vi "table_delete_subtable_item.vi"(7 "subtables":string[](array[string]), 8 "error in (no error)":errorcluster, 10 "subkeys":string[](array[string]), 11 "Table in":refnum<class "Table.lvclass">) -> (0 "error out":errorcluster, 2 "found?":bool, 3 "Table out":refnum<class "Table.lvclass">)   [LabVIEW 2020, in "toml.lvclass"]
uses:
  toml.lvclass
  Table/Table.lvclass
  toml.lvclass/toml.ctl
  Item/Item.lvclass
  InlineTable/InlineTable.lvclass
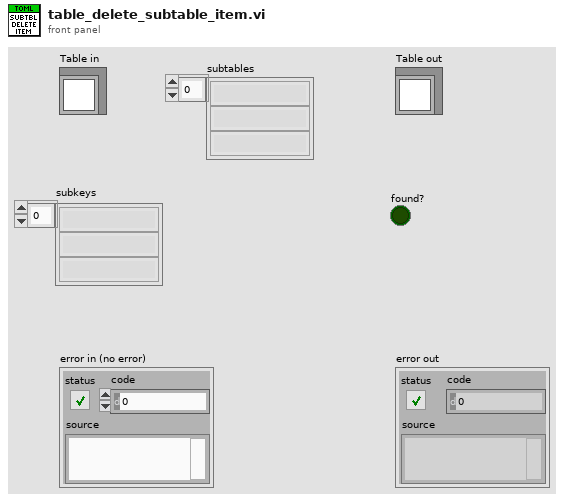
[diagram p1: front panel]
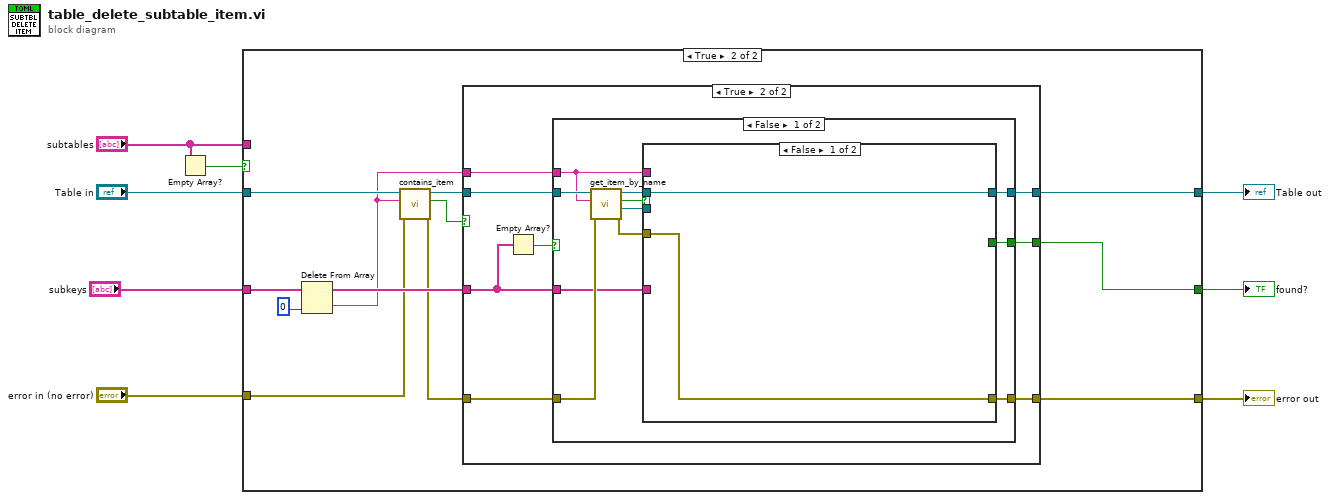
[diagram p0: block diagram]
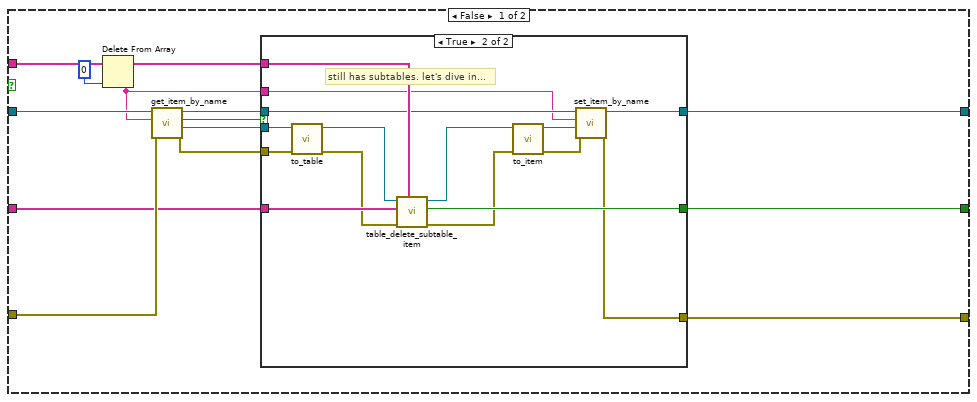
[diagram p2: hidden frame]
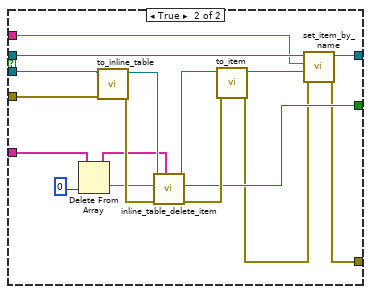
[diagram p5: hidden frame]
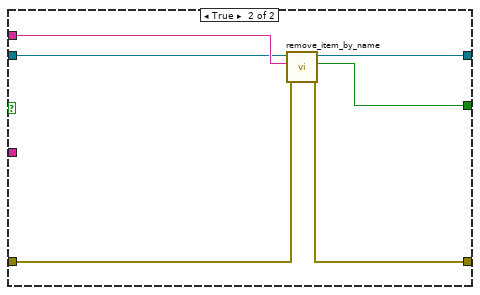
[diagram p6: hidden frame]
diagram:
  n1 = Empty Array?(array="subtables") -> (empty?=w3:bool)
  n2 = case shown="True" w3 {
    tunnel: [w10 w46] -> w8
    tunnel: "subkeys" -> [w15 w49]
    tunnel: [w12 w48] -> w6
    tunnel: "Table in" -> [w19 w44]
    tunnel: "error in (no error)" -> [w18 w42]
    tunnel: "subtables" -> [w22 _]
    tunnel: [w14 w51] -> w1
    frame False {
      n3 = Delete From Array(array=w22, index=0) -> (deleted portion=w11:string, array with subset deleted=w20:string[])  [unwired: 1 in]
      n4 = call "get_item_by_name.vi"("error in (no error)"=w18, "item_name"=w11, "Table in"=w19) -> ("error out"=w16:errorcluster, "Item"=w17:refnum<class "Item.lvclass">, "found?"=w9:bool, "Table out"=w13:refnum<class "Table.lvclass">)  [unwired: 4 in, 1 out]
      n5 = case shown="True" w9 {
        tunnel: w20 -> [_ w39]
        tunnel: w17 -> [_ w38]
        tunnel: w16 -> [w23 w37]
        tunnel: w15 -> [_ w36]
        tunnel: [_ w33] -> w14
        tunnel: w13 -> [w24 w32]
        tunnel: [w24 w31] -> w12
        tunnel: w11 -> [_ w30]
        tunnel: [w23 w25] -> w10
        frame False {
        }
        frame True {
          # "still has subtables. let's dive in..."
          n6 = call "to_table.vi"("error in (no error)"=w37, "Item in"=w38) -> ("error out"=w35:errorcluster, "Table"=w34:refnum<class "Table.lvclass">)  [unwired: 8 in]
          n7 = call "table_delete_subtable_item.vi"("subtables"=w39, "error in (no error)"=w35, "subkeys"=w36, "Table in"=w34) -> ("error out"=w29:errorcluster, "found?"=w33:bool, "Table out"=w28:refnum<class "Table.lvclass">)  [unwired: 5 in]
          n8 = call "to_item.vi"("error in (no error)"=w29, "Table in"=w28) -> ("error out"=w26:errorcluster, "Item out"=w27:refnum<class "Item.lvclass">)  [unwired: 8 in]
          n9 = call "set_item_by_name.vi"("error in (no error)"=w26, "Item"=w27, "item_name"=w30, "Table in"=w32) -> ("error out"=w25:errorcluster, "Table out"=w31:refnum<class "Table.lvclass">)  [unwired: 6 in]
        }
      }
    }
    frame True {
      n10 = Delete From Array(array=w49, index=0) -> (deleted portion=w40:string, array with subset deleted=w47:string[])  [unwired: 1 in]
      n11 = call "contains_item.vi"("error in (no error)"=w42, "item_name"=w40, "Table in"=w44) -> ("error out"=w43:errorcluster, "contains_item"=w41:bool, "Table out"=w45:refnum<class "Table.lvclass">)  [unwired: 6 in]
      n12 = case shown="True" w41 {
        tunnel: [_ w56] -> w51
        tunnel: w40 -> [_ w61]
        tunnel: [w52 w60] -> w48
        tunnel: w47 -> [_ w54]
        tunnel: [w53 w59] -> w46
        tunnel: w45 -> [w52 w58]
        tunnel: w43 -> [w53 w57]
        frame False {
        }
        frame True {
          n13 = Empty Array?(array=w54) -> (empty?=w55:bool)
          n14 = case shown="False" w55 {
            tunnel: w61 -> [w68 w97]
            tunnel: [w67 w96] -> w60
            tunnel: [w63 w95] -> w59
            tunnel: w58 -> [w72 w94]
            tunnel: w57 -> [w66 w93]
            tunnel: [w64 w92] -> w56
            tunnel: w54 -> [w65 _]
            frame False {
              n15 = call "get_item_by_name.vi"("error in (no error)"=w66, "item_name"=w68, "Table in"=w72) -> ("error out"=w70:errorcluster, "Item"=w71:refnum<class "Item.lvclass">, "found?"=w62:bool, "Table out"=w69:refnum<class "Table.lvclass">)  [unwired: 4 in, 1 out]
              n16 = case shown="False" w62 {
                tunnel: w71 -> [_ w91]
                tunnel: w70 -> [w73 w90]
                tunnel: w69 -> [w74 w89]
                tunnel: w68 -> [_ w88]
                tunnel: [w74 w87] -> w67
                tunnel: w65 -> [_ w78]
                tunnel: [_ w77] -> w64
                tunnel: [w73 w75] -> w63
                frame False {
                }
                frame True {
                  n17 = Delete From Array(array=w78, index=0) -> (deleted portion=w80:string, array with subset deleted=w79:string[])  [unwired: 1 in]
                  n18 = call "to_inline_table.vi"("error in (no error)"=w90, "Item in"=w91) -> ("error out"=w85:errorcluster, "InlineTable"=w83:refnum<class "InlineTable.lvclass">)  [unwired: 8 in]
                  n19 = call "inline_table_delete_item.vi"("subtables"=w79, "error in (no error)"=w85, "key"=w80, "InlineTable in"=w83) -> ("error out"=w84:errorcluster, "removed?"=w77:bool, "InlineTable out"=w82:refnum<class "InlineTable.lvclass">)  [unwired: 5 in]
                  n20 = call "to_item.vi"("error in (no error)"=w84, "Table in"=w82) -> ("error out"=w76:errorcluster, "Item out"=w86:refnum<class "Item.lvclass">)  [unwired: 8 in]
                  n21 = call "set_item_by_name.vi"("error in (no error)"=w76, "Item"=w86, "item_name"=w88, "Table in"=w89) -> ("error out"=w75:errorcluster, "Table out"=w87:refnum<class "Table.lvclass">)  [unwired: 6 in]
                }
              }
            }
            frame True {
              n22 = call "remove_item_by_name.vi"("error in (no error)"=w93, "item_name"=w97, "Table in"=w94) -> ("error out"=w95:errorcluster, "removed?"=w92:bool, "Table out"=w96:refnum<class "Table.lvclass">)  [unwired: 6 in]
            }
          }
        }
      }
    }
  }
  "error out" <- w8
  "Table out" <- w6
  "found?" <- w1
